vi "Configure EN-DC LTE.vi"(7 "Carrier Position (Left)":i32(ring) items=["Left", "Right"], 8 "error in (no error)":errorcluster, 9 "Bandwidth (5 MHz)":i32(ring) items=["5 MHz", "10 MHz", "15 MHz", "20 MHz", "25 MHz", "30 MHz", "40 MHz", "50 MHz", "60 MHz", "80 MHz", "90 MHz", "100 MHz"], 10 "Instance (1)":T1=1, 11 "VISA resource name":refnum<visa-resource-name>) -> (0 "error out":errorcluster, 3 "VISA resource name out":refnum<visa-resource-name>)   [LabVIEW 2020, in "Rohde&Schwarz CMWXP NR FR1 Measurement.lvlib"]
doc: "Configures LTE settings for EN-DC.\n\nAttribute:\nRSCMWXPNRFR1M_ATTR_EN_DC_LTE\n\nRemote-control command:\nCONFigure:NRSub:MEAS<i>:MEValuation:ENDC:EUTRa"
uses:
  <instrlib>/Rohde&Schwarz CMWXP NR FR1 Measurement/Rohde&Schwarz CMWXP NR FR1 Measurement.lvlib
  <instrlib>/Rohde&Schwarz CMWXP NR FR1 Measurement/Private/_Instance.ctl
  <instrlib>/Rohde&Schwarz CMWXP NR FR1 Measurement/Private/rsidr_core.llb/rsidr_core.lvlib
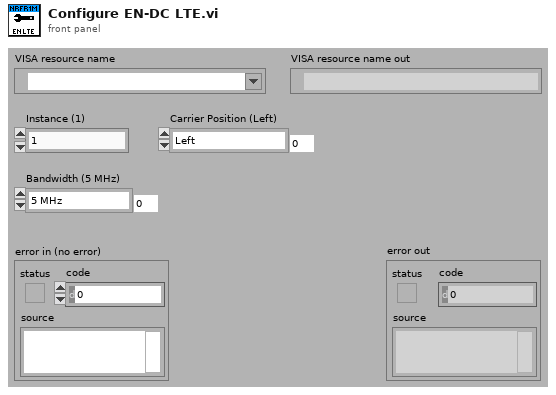
[diagram p1: front panel]
types:
  T1 = typedef "Rohde&Schwarz CMWXP NR FR1 Measurement.lvlib/_Instance.ctl" = i32
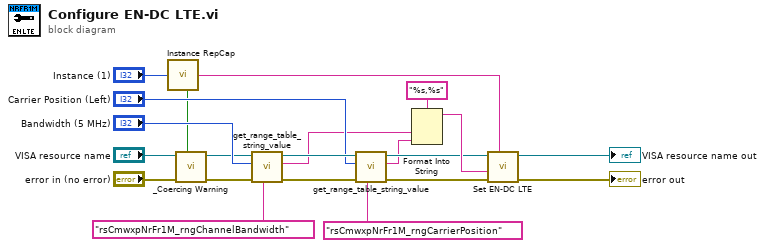
[diagram p0: block diagram]
diagram:
  n1 = call <instrlib>:"Instance RepCap.vi"("Instance In"="Instance (1)") -> ("In Range?"=w5:bool, "RepCap Identifier Out"=w20:string)  [unwired: 1 in]
  n2 = call <instrlib>:"_Coercing Warning.vi"("In Range?"=w5, "error in (no error)"="error in (no error)", "VISA resource name"="VISA resource name") -> ("error out"=w2:errorcluster, "VISA resource name out"=w1:refnum<visa-resource-name>)  [unwired: 7 in]
  n3 = call <instrlib>:"get_range_table_string_value.vi"("Range Table ID in"="rsCmwxpNrFr1M_rngChannelBandwidth", "error in"=w2, "I32 input"="Bandwidth (5 MHz)", "VISA resource name"=w1) -> ("error out"=w17:errorcluster, "String Value out"=w7:string, "VISA resource name out"=w16:refnum<visa-resource-name>)  [unwired: 5 in]
  n4 = call <instrlib>:"get_range_table_string_value.vi"("Range Table ID in"="rsCmwxpNrFr1M_rngCarrierPosition", "error in"=w17, "I32 input"="Carrier Position (Left)", "VISA resource name"=w16) -> ("error out"=w15:errorcluster, "String Value out"=w6:string, "VISA resource name out"=w12:refnum<visa-resource-name>)  [unwired: 5 in]
  n5 = Format Into String(format string="%s,%s", w7, w6) -> (resulting string=w18:string)  [unwired: 2 in, 1 out]
  n6 = call "Set EN-DC LTE"("Repeated Capabilities"=w20, "error in (no error)"=w15, "EN-DC LTE ()"=w18, "instrument handle"=w12) -> ("error out"=→"error out":errorcluster, "instrument handle out"=→"VISA resource name out":refnum<visa-resource-name>)  [unwired: 6 in]
